vi "ShowOKNGpaticle.vi"(7 "XY差异(新坐标系中)":cluster{dbl, dbl}[](array[cluster]), 8 "Y规格":dbl, 9 "X规格":dbl, 10 "坐标数组":cluster{"P_X":i32, "P_Y":i32}[](array[cluster]), 11 "引用句柄输入":T1) -> (2 "总结果":bool, 3 "结果数组":bool[](array[boolean]))   [LabVIEW 2014]
uses:
  <vilib>/vision/Image Controls.llb/IMAQ Image.ctl
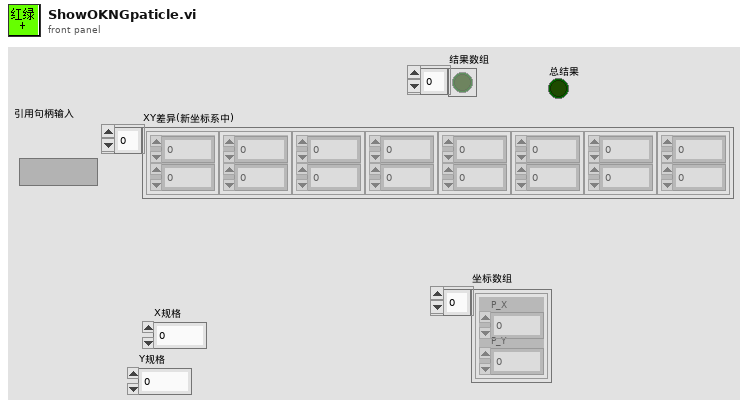
[diagram p1: front panel]
types:
  T1 = typedef "IMAQ Image.ctl" = refnum<image>
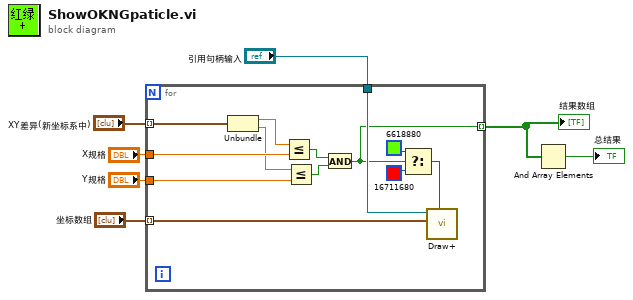
[diagram p0: block diagram]
diagram:
  n1 = for {
    tunnel: "XY差异(新坐标系中)" -> [w10] mode=indexing
    tunnel: "引用句柄输入" -> [w20]
    tunnel: "X规格" -> [w16]
    tunnel: "Y规格" -> [w13]
    tunnel: "坐标数组" -> [w9] mode=indexing
    tunnel: [w8] -> w2 mode=indexing
    n2 = Unbundle(w10) -> (w15:dbl, w14:dbl)
    n3 = Less Or Equal?(x=w15, y=w16) -> (x <= y?=w12:bool)
    n4 = Less Or Equal?(x=w14, y=w13) -> (x <= y?=w11:bool)
    n5 = And(x=w12, y=w11) -> (x .and. y?=w8:bool)
    n6 = Select(t=u32 6618880 ("Color"), s=w8, f=u32 16711680 ("Color")) -> (s? t:f=w19:u32)
    n7 = call "Draw+.vi"("Color"=w19, "input cluster"=w9, "Image In"=w20) -> ()  [unwired: 3 in, 1 out]
  }
  "结果数组" <- w2
  n8 = And Array Elements(Boolean array=w2) -> (logical AND=→"总结果":bool)
